vi "GetType.vi"(8 "error in (no error)":errorcluster, 11 "Disable All Sparse Markers [SM] Msg":refnum<class "Disable All Sparse Markers [SM] Msg.lvclass">) -> (0 "error out":errorcluster, 2 "Data Sample":variant, 3 "Disable All Sparse Markers [SM] Msg":refnum<class "Disable All Sparse Markers [SM] Msg.lvclass">)   [LabVIEW 2015, in "CS++Fgen.lvlib" / "Disable All Sparse Markers [SM] Msg.lvclass"]
doc: "This VI delivers a sample of the data type format the message expects."
uses:
  Disable All Sparse Markers [SM] Msg.lvclass
  Disable All Sparse Markers [SM] Msg.lvclass/Disable All Sparse Markers [SM] Msg.ctl
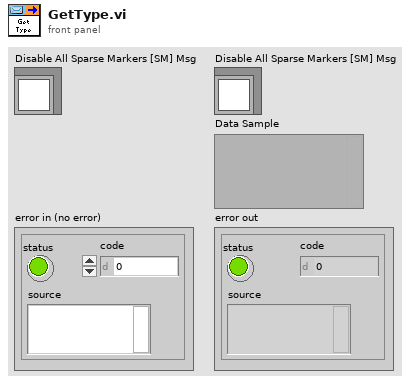
[diagram p1: front panel]
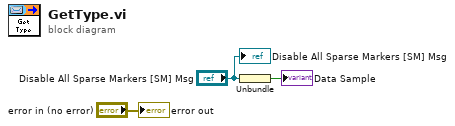
[diagram p0: block diagram]
diagram:
  n1 = Unbundle("Disable All Sparse Markers [SM] Msg") -> (→"Data Sample":bool)
  "error out" <- "error in (no error)"
  "Disable All Sparse Markers [SM] Msg" <- "Disable All Sparse Markers [SM] Msg"
